vi "View CW and Write Judgement.vi"() -> ()   [LabVIEW 2020]
uses:
  Labview Library/Libraries/Basic Experiment/CW Fit Frequency.ctl
  Labview Library/Libraries/Basic Experiment/CW settings.ctl
  Labview Library/Libraries/LaoJi/UT_Utilities/Utilities.lvlib
  Labview Library/Libraries/Basic Experiment/Basic Experiment.lvlib
  Labview Library/Libraries/Color Center Repository/Libraries/Repository Control/Repository Control.lvlib
panel:
  in  "Folder Path":path
  out "CW":T1(graph)=[{"Fre sequence"=[1350.0, 1351.6666666666667, 1353.3333333333333, 1355.0, 1356.6666666666667, 1358.3333333333333, 1360.0, 1361.6666666666667, 1363.3333333333333, 1365.0, 1366.6666666666667, 1368.3333333333333, 1370.0, 1371.6666666666667, 1373.3333333333333, 1375.0, 1376.6666666666667, 1378.3333333333333, 1380.0, 1381.6666666666667, 1383.3333333333333, 1385.0, 1386.6666666666667, 1388.3333333333333, 1390.0, 1391.6666666666667, 1393.3333333333333, 1395.0, 1396.6666666666667, 1398.3333333333333, 1400.0], "Pro Array"=[0.023576918066953237, -0.0017480281389895545, -0.007263715604170227, -0.003638698630136986, -0.004441217918606141, -0.011703176576499335, -0.033005677484958904, -0.009671179883945842, -0.026188455008488966, -0.046696221237069874, -0.033329043881096386, -0.031275649056114734, -0.057291215923842495, -0.07413808001382528, -0.09635672489642506, -0.10355751530459352, -0.08496202099513528, -0.06363636363636363, -0.04259915320141709, -0.03029136182774997, -0.028735632183908046, 0.0027938964109176876, -0.015497553017944535, -0.02762105263157895, -0.01327134404057481, 0.005625456263151115, 0.001029336078229542, -0.005610575083946105, -0.006010486380493627, -0.010508919869485996, 0.01442328268778087]}, {"Fre sequence"=array[301 elements], "Pro Array"=array[301 elements]}]
  out "Pro Array":dbl[](array[numeric])=[0.023576918066953237, -0.0017480281389895545, -0.007263715604170227, -0.003638698630136986, -0.004441217918606141, -0.011703176576499335, -0.033005677484958904, -0.009671179883945842, -0.026188455008488966, -0.046696221237069874, -0.033329043881096386, -0.031275649056114734, -0.057291215923842495, -0.07413808001382528, -0.09635672489642506, -0.10355751530459352, -0.08496202099513528, -0.06363636363636363, -0.04259915320141709, -0.03029136182774997, -0.028735632183908046, 0.0027938964109176876, -0.015497553017944535, -0.02762105263157895, -0.01327134404057481, 0.005625456263151115, 0.001029336078229542, -0.005610575083946105, -0.006010486380493627, -0.010508919869485996, 0.01442328268778087]
  in  "Settings":T2={"Num Pts"=30, "Start freq"=1350.0, "Stop freq"=1400.0, " dBm"=-14.0, "Loop times"=20000, "Ratio Thre(abs)"=0.06, "AutoTrace Before Exp"=TRUE, "RepoSave"=FALSE}
  out "Fre sequence":dbl[](array[numeric])=[1350.0, 1351.6666666666667, 1353.3333333333333, 1355.0, 1356.6666666666667, 1358.3333333333333, 1360.0, 1361.6666666666667, 1363.3333333333333, 1365.0, 1366.6666666666667, 1368.3333333333333, 1370.0, 1371.6666666666667, 1373.3333333333333, 1375.0, 1376.6666666666667, 1378.3333333333333, 1380.0, 1381.6666666666667, 1383.3333333333333, 1385.0, 1386.6666666666667, 1388.3333333333333, 1390.0, 1391.6666666666667, 1393.3333333333333, 1395.0, 1396.6666666666667, 1398.3333333333333, 1400.0]
  out "Fit Frequency":T3={"Fre2"={"Amplitude"=nan, "Position"=nan, "Width"=nan}, "Fre1"={"Amplitude"=-0.1025002919574418, "Position"=1374.3259241492356, "Width"=5.5456538540315705}, "Fre3"={"Amplitude"=nan, "Position"=nan, "Width"=nan}}
  out "Is NV?":bool=TRUE
  in  "Peak Number Limit (10)":i32=10
  # "CW Settings"
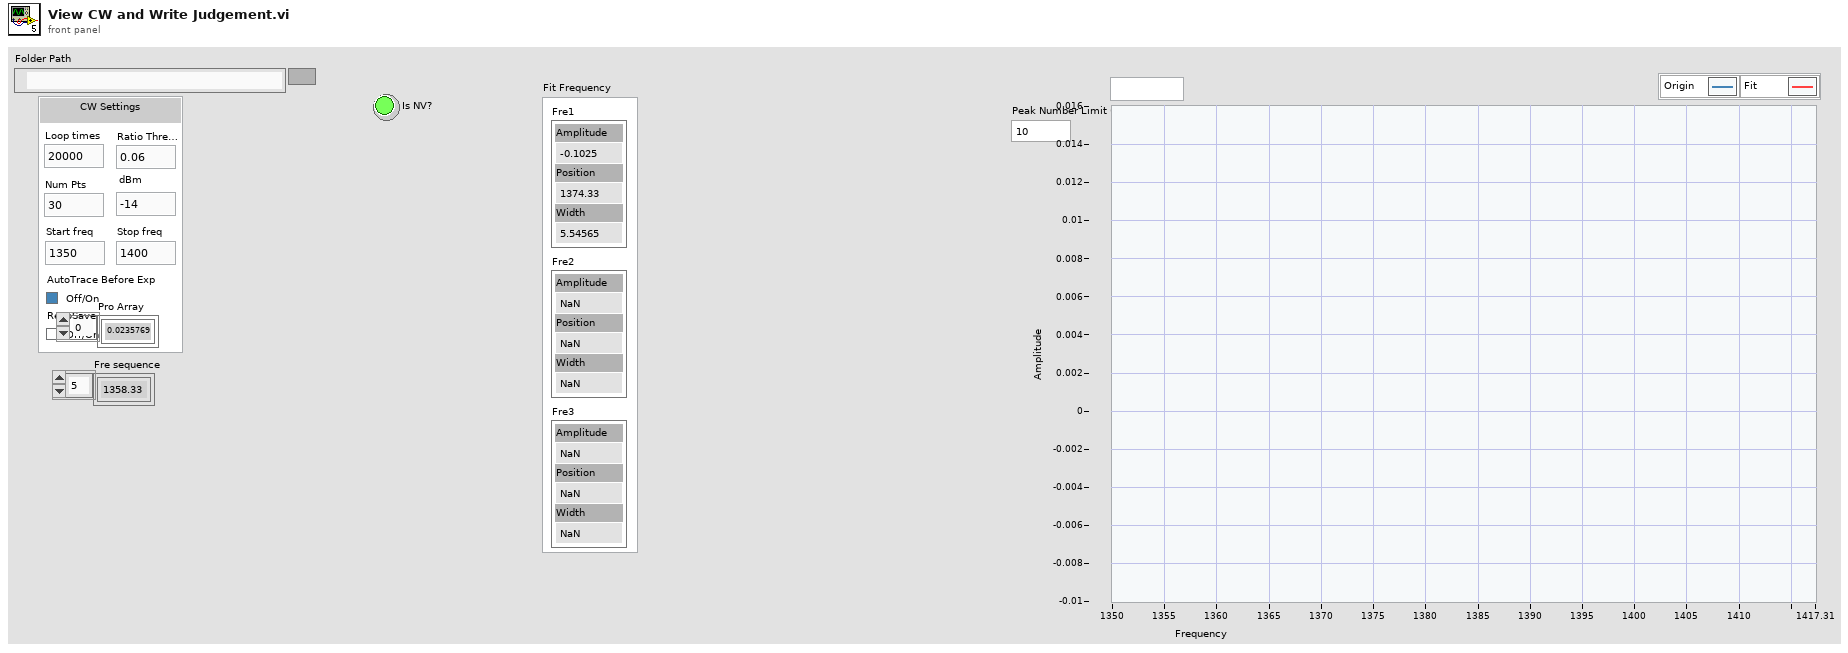
[diagram p1: front panel]
types:
  T1 = cluster{"Fre sequence":dbl[], "Pro Array":dbl[]}[]
  T2 = typedef "Basic Experiment.lvlib/CW settings.ctl" = cluster{"Num Pts":i32, "Start freq":dbl, "Stop freq":dbl, " dBm":dbl, "Loop times":i32, "Ratio Thre(abs)":dbl, "AutoTrace Before Exp":bool, "RepoSave":bool}
  T3 = typedef "Basic Experiment.lvlib/CW Fit Frequency.ctl" = cluster{"Fre2":cluster{"Amplitude":dbl, "Position":dbl, "Width":dbl}, "Fre1":cluster{"Amplitude":dbl, "Position":dbl, "Width":dbl}, "Fre3":cluster{"Amplitude":dbl, "Position":dbl, "Width":dbl}}
  T4 = cluster{"output array":dbl[], "Fre sequence":dbl[]}
  T5 = typedef "Utilities.lvlib/Lorentizan Fit Parameter.ctl" = cluster{"Background":dbl, "Peaks Parameter":T6[]}
  T6 = typedef "Utilities.lvlib/Peak Parameter.ctl" = cluster{"Amplitude":dbl, "Position":dbl, "Width":dbl}
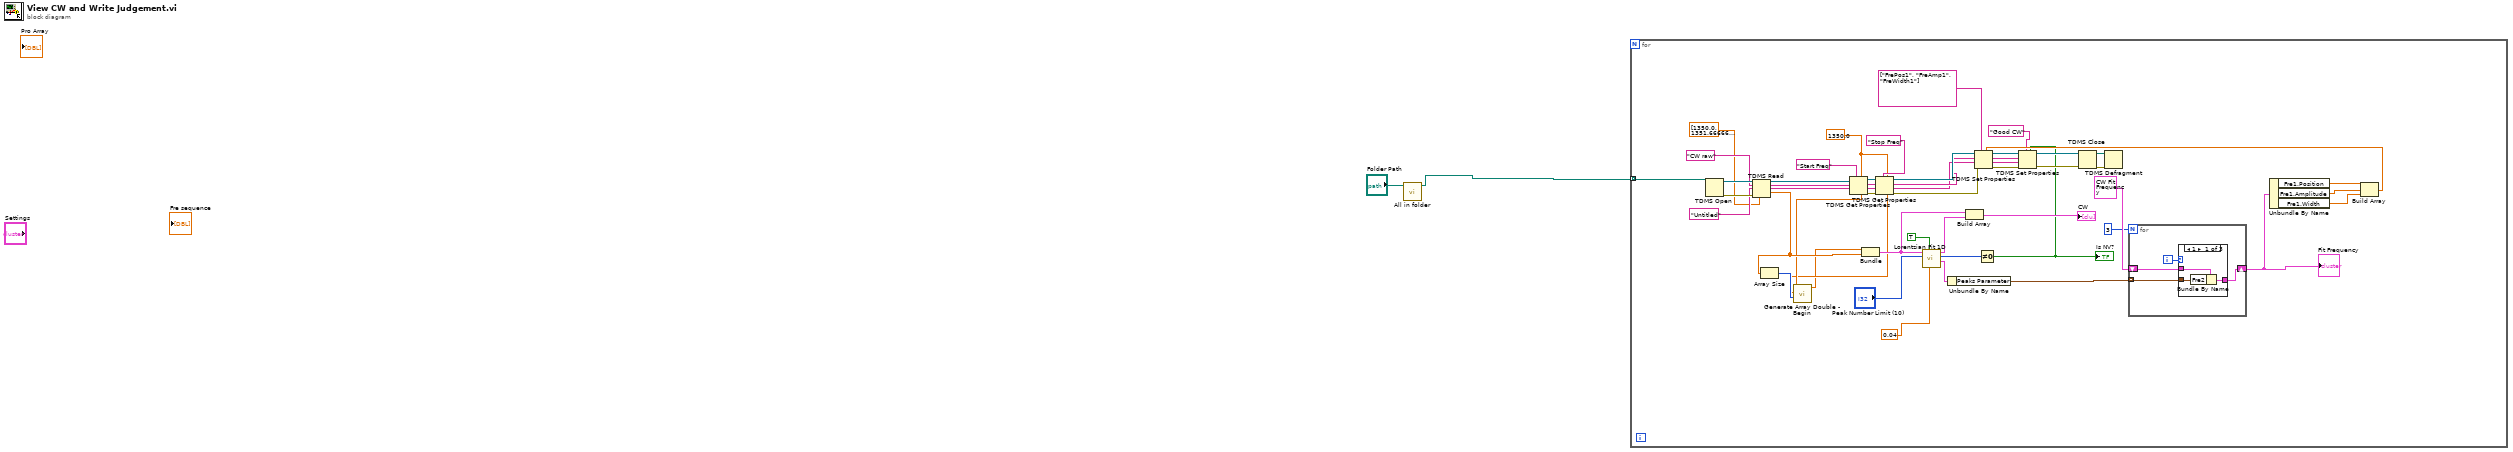
[diagram p0: block diagram]
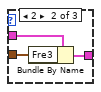
[diagram p2: hidden frame]
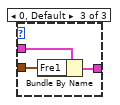
[diagram p3: hidden frame]
diagram:
  n1 = call "All in folder.vi"("Folder Path"="Folder Path") -> ("Tdms list"=w2:path[])  [unwired: 9 in, 1 out]
  n2 = for {
    tunnel: w2 -> [w11] mode=indexing
    w29 = 1350.0
    n3 = TDMS Open(11:w11) -> (0:w42:errorcluster, 3:w43:refnum<k34>)  [unwired: 6 in]
    n4 = TDMS Read(0:w43, 5:"CW raw", 7:"Untitled", 11:w42, 12:dbl[] [1350.0, 1351.6666666666667, 1353.3333333333333, 1355.0, 1356.6666666666667, 1358.3333333333333, 1360.0, 1361.6666666666667, 1363.3333333333333, 1365.0, 1366.6666666666667, 1368.3333333333333, 1370.0, 1371.6666666666667, 1373.3333333333333, 1375.0, 1376.6666666666667, 1378.3333333333333, 1380.0, 1381.6666666666667, 1383.3333333333333, 1385.0, 1386.6666666666667, 1388.3333333333333, 1390.0, 1391.6666666666667, 1393.3333333333333, 1395.0, 1396.6666666666667, 1398.3333333333333, 1400.0] ("Fre sequence")) -> (4:w38:refnum<k34>, 6:w37:string, 8:w36:string, 10:w28:dbl[])  [unwired: 3 in, 2 out]
    n5 = Array Size(array=w28) -> (size(s)=w27:i32)
    n6 = TDMS Get Properties(5:w29, 7:"Start Freq", 9:w36, 10:w37, 11:w38) -> (0:w34:errorcluster, 1:w33:string, 2:w32:string, 3:w31:refnum<k34>, 4:w26:dbl)  [unwired: 1 in, 1 out]
    n7 = TDMS Get Properties(5:w29, 7:"Stop Freq", 8:w34, 9:w33, 10:w32, 11:w31) -> (0:w22:errorcluster, 1:w20:string, 2:w21:string, 3:w23:refnum<k34>, 4:w25:dbl)  [unwired: 1 out]
    n8 = call "Generate Array Double - Begin.vi"("num of step"=w27, "end"=w25, "begin"=w26) -> ("output array"=w24:dbl[])  [unwired: 5 in, 3 out]
    n9 = Bundle("output array"=w24, "Fre sequence"=w28) -> (w51:T4)  [unwired: 1 in]
    n10 = call "Lorentzian Fit 1D.vi"("Amplitude Limit (0.05)"=0.04, "Reverse Peak?"=TRUE, "Peak Number Limit (10)"="Peak Number Limit (10)", "Data"=w51) -> ("Best Fit Parameter"=w50:T5, "Num of Peak Found"=w49:i32, "Fit Result"=w52:cluster{"x":dbl[], "y":dbl[]})  [unwired: 3 in, 2 out]
    n11 = Unbundle By Name(w50) -> ("Peaks Parameter"=w48:T6[])
    n12 = Build Array(w51, w52) -> (→"CW":cluster{"x":dbl[], "y":dbl[]}[])
    n13 = Not Equal To 0?(x=w49) -> (x != 0?=w5:bool)
    "Is NV?" <- w5
    n14 = for {
      N: 3 -> [_]
      tunnel: w48 -> [w56] mode=indexing
      shift-right: [w55] -> w18
      shift-left: T3 {"Fre2"={"Amplitude"=nan, "Position"=nan, "Width"=nan}, "Fre1"={"Amplitude"=nan, "Position"=nan, "Width"=nan}, "Fre3"={"Amplitude"=nan, "Position"=nan, "Width"=nan}} ("Fit Frequency") -> [w58]
      i -> [w57]
      n15 = case shown="1" w57 {
        tunnel: w58 -> [w61 w64 w67]
        tunnel: w56 -> [w60 w63 w66]
        tunnel: [w59 w62 w65] -> w55
        frame 1 {
          n16 = Bundle By Name(cluster=w61, "Fre2"=w60) -> (w59:T3)
        }
        frame 2 {
          n17 = Bundle By Name(cluster=w64, "Fre3"=w63) -> (w62:T3)
        }
        frame 0, Default {
          n18 = Bundle By Name(cluster=w67, "Fre1"=w66) -> (w65:T3)
        }
      }
    }
    "Fit Frequency" <- w18
    n19 = Unbundle By Name(w18) -> ("Fre1.Position"=w17:dbl, "Fre1.Amplitude"=w16:dbl, "Fre1.Width"=w15:dbl)
    n20 = Build Array(w17, w16, w15) -> (w14:dbl[])
    n21 = TDMS Set Properties(5:w14, 7:string[] ["FrePos1", "FreAmp1", "FreWidth1"] ("property names"), 8:w22, 9:w20, 10:w21, 11:w23) -> (0:w10:errorcluster, 1:w3:string, 2:w4:string, 3:w8:refnum<k34>)
    n22 = TDMS Set Properties(5:w5, 7:"Good CW", 8:w10, 9:w3, 10:w4, 11:w8) -> (0:w9:errorcluster, 3:w7:refnum<k34>)  [unwired: 2 out]
    n23 = TDMS Close(8:w9, 11:w7) -> (0:w13:errorcluster, 3:w12:path)
    n24 = TDMS Defragment(4:w13, 7:w12) -> ()  [unwired: 1 out]
  }
